vi "enableChannel.vi"(4 "range":dbl, 6 "Enable":bool, 7 "Device Name":string, 8 "error in (no error)":errorcluster, 9 "Channel (0.1.2.3)":string, 11 "Refnum in":refnum<k21>) -> (0 "error out":errorcluster, 3 "Refnum out":refnum<k21>)   [LabVIEW 2011]
panel:
  out "Enabled (array)":bool[](array[boolean])=[FALSE, TRUE, TRUE, TRUE]
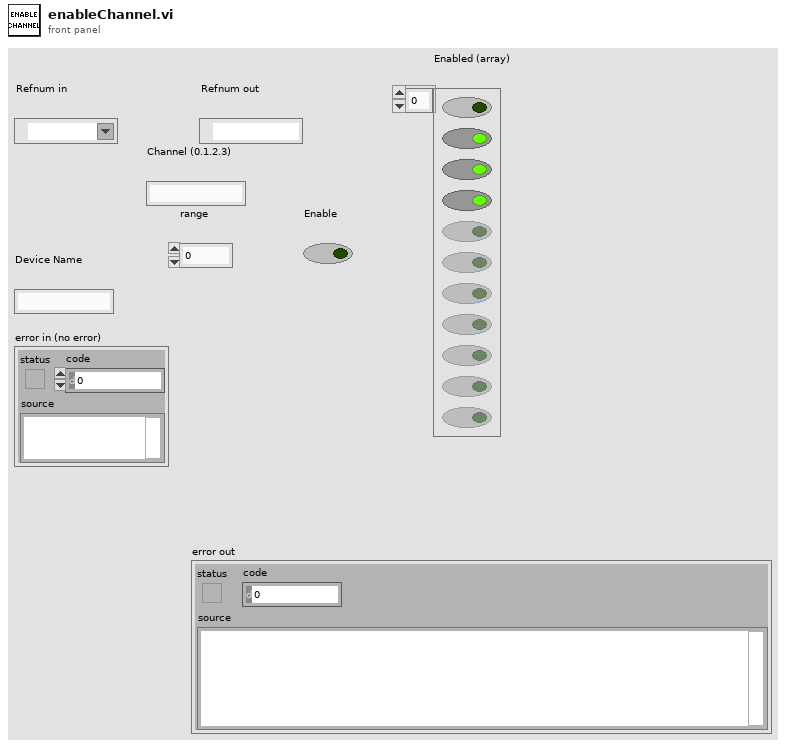
[diagram p1: front panel]
types:
  T1 = typedef "OnOffTypeDef.ctl" = enum16{"off", "on"}
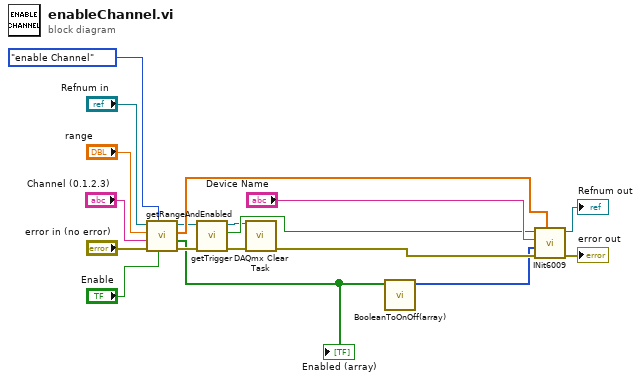
[diagram p0: block diagram]
diagram:
  n1 = call "getRangeAndEnabled.vi"("Enable"="Enable", "mode"=enum16{"enable Channel", "get/set Range"}."enable Channel", "error in (no error)"="error in (no error)", "Channel (0.1.2.3)"="Channel (0.1.2.3)", "range (V)"="range", "Refnum in"="Refnum in") -> ("error out"=w17:errorcluster, "Enabled (array)"=w2:bool[], "Range"=w18:dbl[], "Refnum out"=w15:refnum<k21>)  [unwired: 2 in]
  "Enabled (array)" <- w2
  n2 = call "getTrigger.vi"("error in (no error)"=w17, "Refnum in"=w15) -> ("error out"=w13:errorcluster, "triggered"=w11:bool, "Refnum out"=w10:refnum<k21>)  [unwired: 7 in]
  n3 = call "DAQmx Clear Task.vi"("task in"=w10, "error in"=w13) -> ("error out"=w7:errorcluster)  [unwired: 13 in]
  n4 = call "BooleanToOnOff(array).vi"("Enabled (array)"=w2) -> ("Array"=w1:T1[])  [unwired: 10 in]
  n5 = call "INit6009.vi"("Range"=w18, "error in (no error)"=w7, "ChannelEnable"=w1, "DAQmx Device Name"="Device Name", "Trigger"=w11) -> ("error out"=→"error out":errorcluster, "Refnum out"=→"Refnum out":refnum<k21>)  [unwired: 4 in, 1 out]
